vi "Update Washer Records.vi"(0 "GUI Aisle In":T1[](array[typedef]) {"Cycle Count" format="%05d"}, 7 "Dryer Com Info":T3[](array[typedef])) -> (4 "Aisle Array Out":T1[](array[typedef]) {"Cycle Count" format="%05d"})   [LabVIEW 2009]
uses:
  Washer.ctl
  Dryer Wilt/Dryer Details.ctl
  Dryer Wilt/Dryer Com Port Info.ctl
  Dryer Wilt/Dryer Status Ctrl.ctl
  Dryer Wilt/Update Wilt GUI Control.ctl
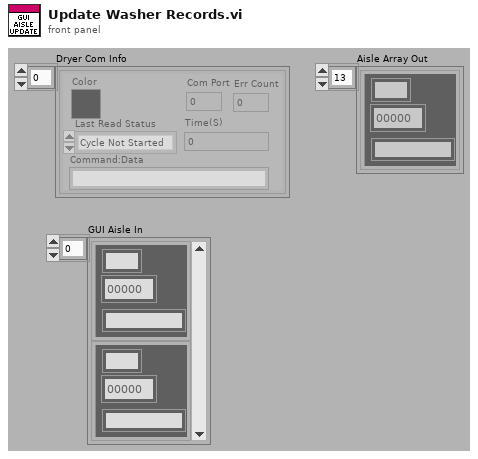
[diagram p1: front panel]
types:
  T1 = typedef "Washer.ctl" = cluster{"Serial Number":string, "Cycle Count":i32, "Station Number":string, "Dryer Details":T2, "Sample Record(t, CC, ASCII, Status ) ":string[], "Hist Record(Cycle Count, t-comp) ":string[][], "Status Color":u32, "Com Port":u8, "Bad Com Count":i32, "Boolean":bool}
  T2 = typedef "Dryer Details.ctl" = cluster{"Station":string, "Cycle Count":string, "Status":string, "Debug ASCII":string, "Notes":string, "File: Current Cycle":string, "Serial Number":string, "Total Time On":string, "TR Number":string, "File: Historic Data":string}
  T3 = typedef "Dryer Com Port Info.ctl" = cluster{"Color":u32, "Last Read Status":T4, "Command:Data":string, "Com Port":u8, "Time(S)":dbl, "Err Count":u8}
  T4 = typedef "Dryer Status Ctrl.ctl" = enum16{"Cycle Not Started", "Cycle Running", "Paused", "Cycle Completed", "Eval Mode Entered", "Err"}
  T5 = typedef "Update Wilt GUI Control.ctl" = enum16{"Init Station Number", "Update Detail Data", "Update Status", "Init Com Port Num", "Update Sample Info"}
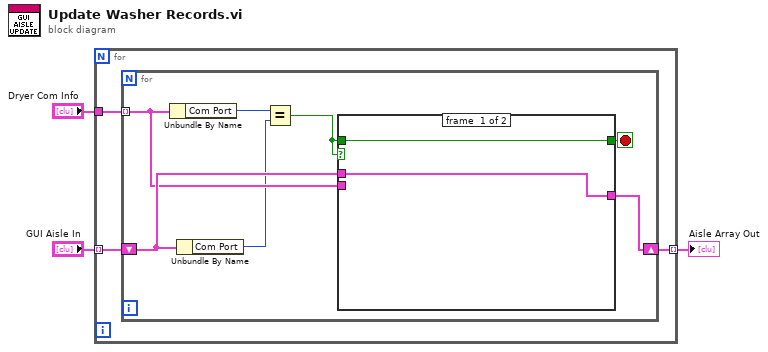
[diagram p0: block diagram]
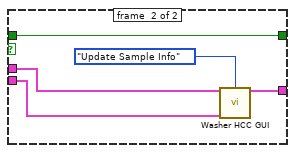
[diagram p2: hidden frame]
diagram:
  n1 = for {
    tunnel: "GUI Aisle In" -> [w6] mode=indexing
    tunnel: "Dryer Com Info" -> [w5]
    tunnel: [w4] -> w3 mode=indexing
    n2 = for {
      tunnel: w5 -> [w10] mode=indexing
      shift-right: [w11] -> w4
      shift-left: w6 -> [w12]
      stop <- w8 stop-if-true
      n3 = Unbundle By Name(w10) -> ("Com Port"=w13:u8)
      n4 = Unbundle By Name(w12) -> ("Com Port"=w9:u8)
      n5 = Equal?(x=w13, y=w9) -> (x = y?=w7:bool)
      n6 = case shown="True" w7 {
        tunnel: w12 -> [w15 w20]
        tunnel: w10 -> [_ w18]
        tunnel: [w15 w19] -> w11
        tunnel: [w14 w16] -> w8
        tunnel: w7 -> [w14 w16]
        frame #0 {
        }
        frame #1 {
          n7 = call "Washer HCC GUI.vi"("Washer In"=w20, "Enum"=Update_Wilt_GUI_Control."Update Sample Info", "Washer Status Serial Data In"=w18) -> ("Washer Out"=w19:T1)  [unwired: 10 in, 2 out]
        }
      }
    }
  }
  "Aisle Array Out" <- w3
